vi "QT_FGClose.vi"(0 "QT Ref In":T1, 5 "error in (no error)":errorcluster, 8 "Private":T2) -> (14 "QT Ref Out":T1, 19 "error out":errorcluster={"status"=TRUE, "code"=-43, "source"=""})   [LabVIEW 2024]
doc: "Create and initilize a new Frame grabber channel"
uses:
  <userlib>/ImageProcessing/QTLIB_2595_LV86/QT_Selector.ctl
  <userlib>/ImageProcessing/QTLIB_2595_LV86/QT_Ref.ctl
  <userlib>/ImageProcessing/QTLIB_2595_LV86/QT_Private.ctl
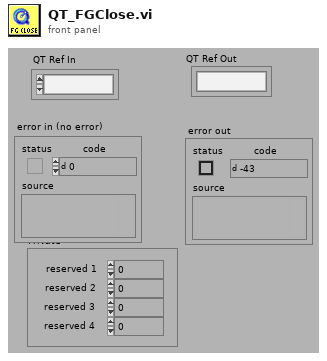
[diagram p1: front panel]
types:
  T1 = typedef "QT_Ref.ctl" = refnum<k1>
  T2 = typedef "QT_Private.ctl" = cluster{"reserved 1":i32, "reserved 2":i32, "reserved 3":i32, "reserved 4":i32}
  T3 = typedef "QT_Selector.ctl" = enum32{"do nothing", "Get all Sources", "Get Source info", "Open Image", "Save Image to File", "Effect", "Close", "SG Grab", "Compress in Memory", "Decompress to Memory", "New Movie", "Open Movie", "Add Frame", "Get Frame", "Close Movie", "Get QT & CIN info", "SG init", "SG Close", "Open sound file", "Close sound file", "Read sound data", "Write sound data", "Import sound", "Export sound", "Add sound to movie", "Get sound from movie", "reserved", "reserved 1", "reserved 2"}
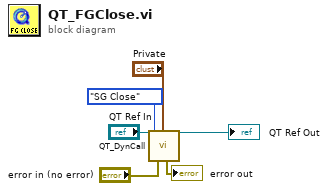
[diagram p0: block diagram]
diagram:
  n1 = call <userlib>:"QT_DynCall.vi"("QT Ref In"="QT Ref In", "error in (no error)"="error in (no error)", "Selector"=QT_Selector."SG Close", "Private"="Private") -> ("QT Ref Out"=→"QT Ref Out":T1, "error out"=→"error out":errorcluster)  [unwired: 8 in, 14 out]
